vi "Read instrT.vi"(8 "error in (no error)":errorcluster, 11 "CPC Data in":refnum<class "CPC Data.lvclass">) -> (0 "error out":errorcluster, 2 "instrT":cluster{"cond T":dbl, "sat T":dbl, "opt T":dbl}, 3 "CPC Data out":refnum<class "CPC Data.lvclass">)   [LabVIEW 2014, in "CPC Data.lvclass"]
uses:
  CPC Data.lvclass
  CPC Data.lvclass/CPC Data.ctl
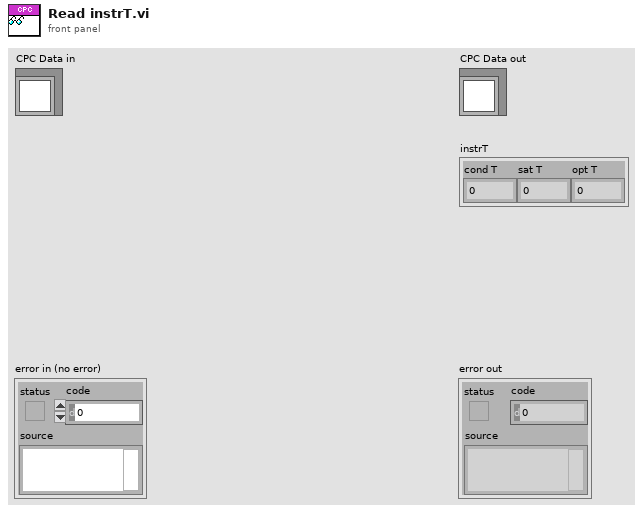
[diagram p1: front panel]
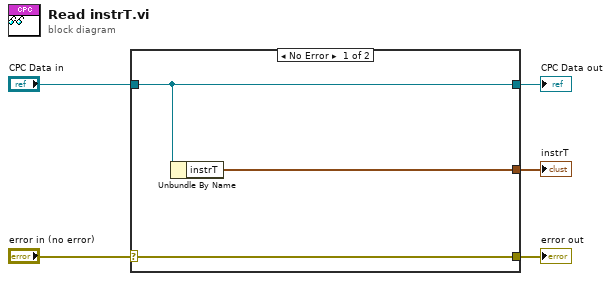
[diagram p0: block diagram]
diagram:
  n1 = case shown="No Error" "error in (no error)" {
    selector: "error in (no error)" -> [w8 w9]
    tunnel: [w8 w9] -> w4
    tunnel: [w7 w10] -> w2
    tunnel: "CPC Data in" -> [w7 w10]
    tunnel: [w6 _] -> w1
    frame No Error {
      n2 = Unbundle By Name(w7) -> ("instrT"=w6:cluster{"cond T":dbl, "sat T":dbl, "opt T":dbl})
    }
    frame Error {
    }
  }
  "error out" <- w4
  "CPC Data out" <- w2
  "instrT" <- w1
